vi "Autonomous Independent.vi"() -> ()   [LabVIEW 2018]
doc: "This VI is called when autonomous begins, and will automatically be terminated when autonomous ends. You can carry out timed or sensor driven robot movement independently without needing to return to the caller."
uses:
  <vilib>/Rock Robotics/WPI/RobotDrive/WPI_RobotDriveArcadeDrive_Standard(NoSaturation).vi
  <vilib>/Rock Robotics/Network Tables/NT Write Numeric Array.vi
  <vilib>/Rock Robotics/WPI/Gyro/WPI_GyroXRS450_SPI_Open.vi
  <vilib>/Rock Robotics/Network Tables/NT Write Number.vi
  <vilib>/Rock Robotics/Network Tables/NT Read String.vi
  <vilib>/Rock Robotics/SystemInterfaces/spilib/spi_bus.ctl
panel:
  out "Ultrasonic 2":dbl
  out "Ultrasonic":dbl
  out "Degrees 2":dbl(knob) scale=0.0..360.0
  out "Degrees":dbl(knob) scale=0.0..360.0
  in  "Reset Angle?":bool
  out "Calibrated?":bool
  out "Degrees":dbl(knob) scale=0.0..360.0
  out "Degrees 2":dbl(knob) scale=0.0..360.0
  in  "SPI Bus":T1
  out "Device Found":bool
  in  "Sample Rate (Hz)":dbl=1000.0 min=50.0 max=20000.0 format="%#_13g"
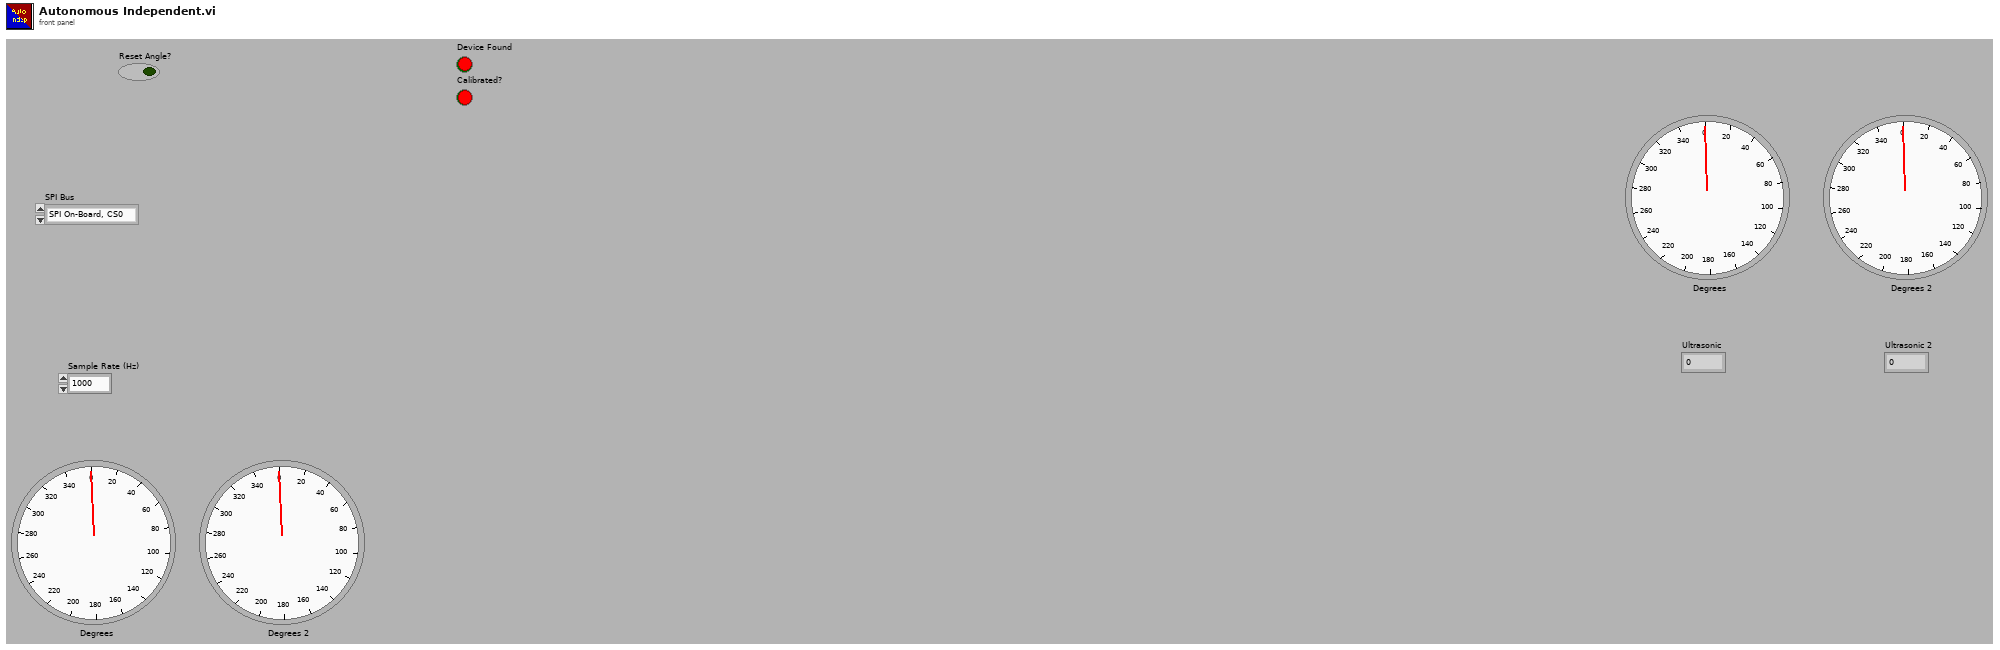
[diagram p1: front panel]
types:
  T1 = typedef "spi_bus.ctl" = enum16{"SPI On-Board, CS0", "SPI On-Board, CS1", "SPI On-Board, CS2", "SPI On-Board, CS3", "SPI MXP", "Invalid"}
  T2 = typedef "WPI_JoystickDevRef.ctl" = cluster{"Device":T3}
  T3 = typedef "WPI_JoystickDeviceEnum.ctl" = enum16{"USB 0", "USB 1", "USB 2", "USB 3", "USB 4", "USB 5"}
  T4 = typedef "WPI_RobotDriveDevRef.ctl" = cluster{"DevStatus":errorcluster, "Motors[]":T5[], "Square Inputs":bool, "Max Output":dbl}
  T5 = typedef "WPI_MotorControlDeviceRef.ctl" = cluster{"DeviceStatus":errorcluster, "Type":T6, "PWM":cluster{"PWM Channel":T7, "DeadBand":T8}, "CAN":cluster{"Device Number":u8, "SetOutput VI Ref":variant, "GetOutput VI Ref":variant, "Enable VI Ref":variant, "Disable VI Ref":variant, "Data":variant}, "Invert":bool, "DIO PWM":cluster{"PWM \"Enable\" Channel":T7, "DIOChannel":T9, "PWM Rate":dbl}}
  T6 = typedef "WPI_MotorControlType.ctl" = enum16{"PWM", "CAN", "DIO PWM"}
  T7 = typedef "FPGA_DIOPWMChannel.ctl" = enum8{"PWM 0", "PWM 1", "PWM 2", "PWM 3", "PWM 4", "PWM 5", "PWM 6", "PWM 7", "PWM 8", "PWM 9", "PWM MXP 0", "PWM MXP 1", "PWM MXP 2", "PWM MXP 3", "PWM MXP 4", "PWM MXP 5", "PWM MXP 6", "PWM MXP 7", "PWM MXP 8", "PWM MXP 9", "Invalid"}
  T8 = typedef "WPI_PWMDeadband.ctl" = cluster{"Name":string, "maxPositivePwm":i32, "minPositivePwm":i32, "centerPwm":i32, "maxNegativePwm":i32, "minNegativePwm":i32, "angularRange":u16}
  T9 = typedef "FPGA_DIOChannel.ctl" = enum8{"DIO 0", "DIO 1", "DIO 2", "DIO 3", "DIO 4", "DIO 5", "DIO 6", "DIO 7", "DIO 8", "DIO 9", "DIO MXP 0", "DIO MXP 1", "DIO MXP 2", "DIO MXP 3", "DIO MXP 4", "DIO MXP 5", "DIO MXP 6", "DIO MXP 7", "DIO MXP 8", "DIO MXP 9", "DIO MXP 10", "DIO MXP 11", "DIO MXP 12", "DIO MXP 13", "DIO MXP 14", "DIO MXP 15", "SPI Port CS1", "SPI Port CS2", "SPI Port CS3", "SPI Port MISO", "SPI Port MOSI", "Invalid"}
  T10 = typedef "WPI_GyroDevRef.ctl" = cluster{"DevStatus":errorcluster, "Analog Channel":T11, "Gain (VoltsPerDegree/Second)":dbl, "Gyro Type":enum16{"Analog", "XRS450"}, "Handle":i32, "SPI Bus":T1, "Device Found":bool, "Sample Rate":dbl, "Calibrate On Open":bool, "Offset":dbl}
  T11 = typedef "FPGA_AIChannel.ctl" = enum8{"AI 0", "AI 1", "AI 2", "AI 3", "AI MXP 0", "AI MXP 1", "AI MXP 2", "AI MXP 3", "Invalid"}
  T12 = typedef "WPI_AnalogChannelDevRef.ctl" = cluster{"DevStatus":errorcluster, "Analog Channel":T11}
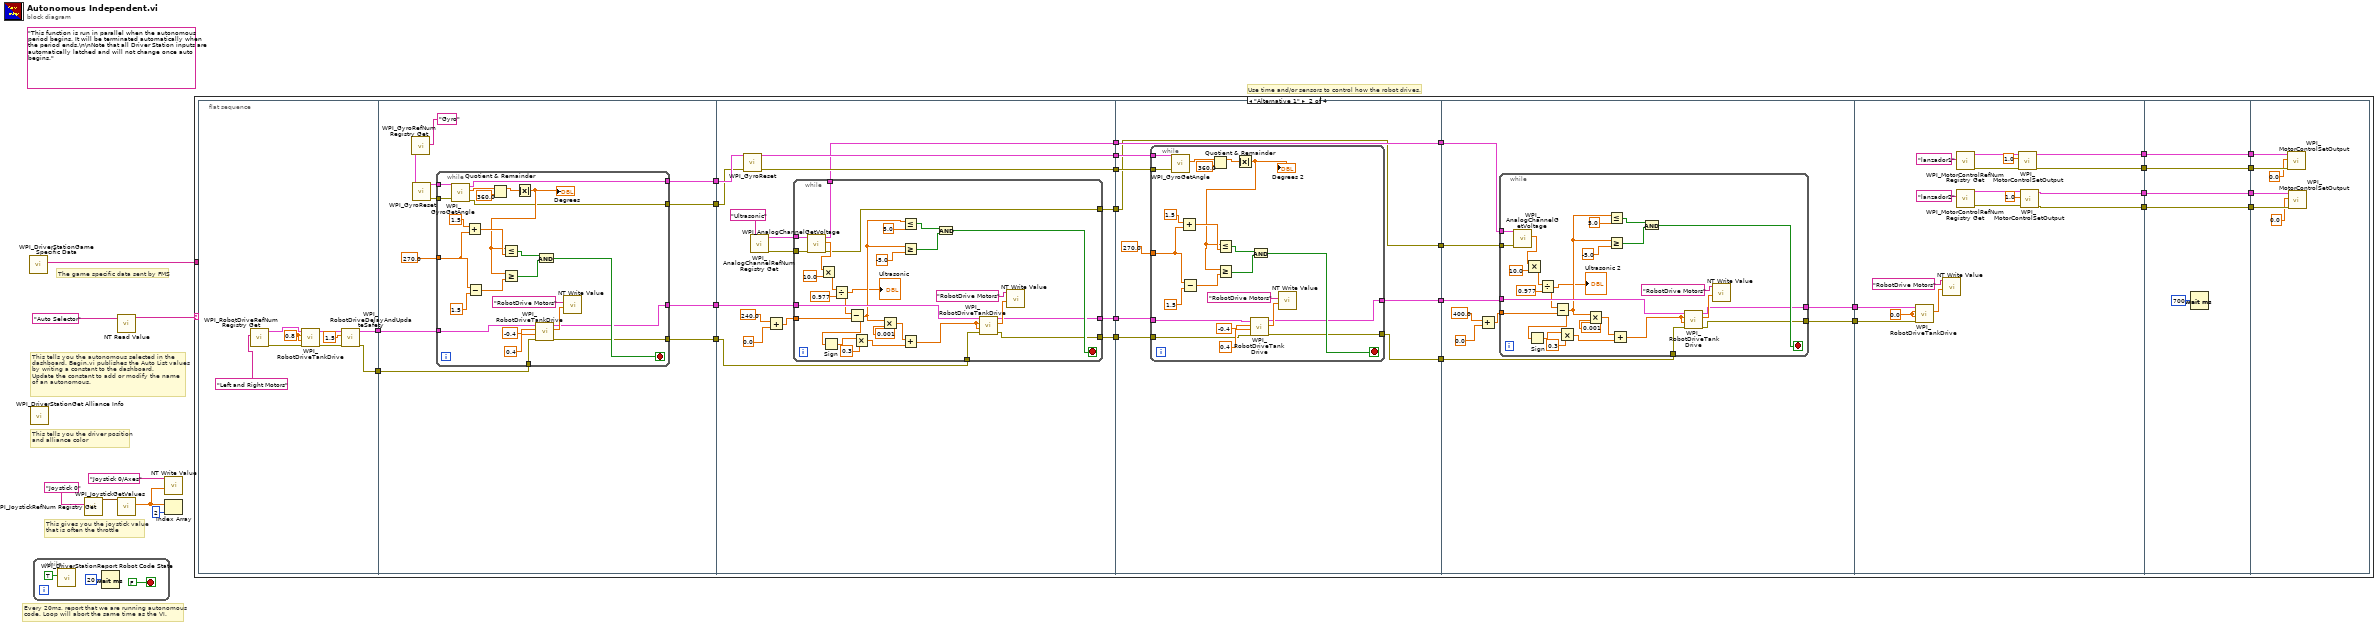
[diagram p0: block diagram]
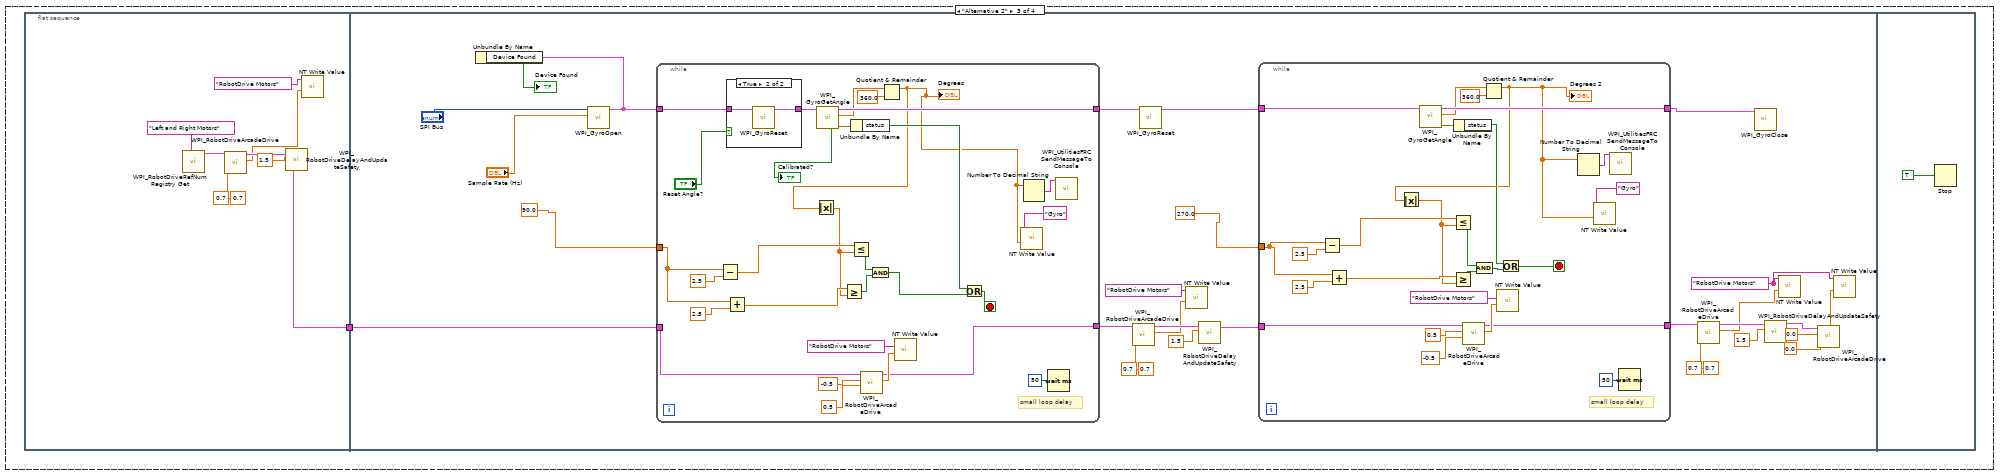
[diagram p3: hidden frame]
diagram:
  (unwired) "This function is run in parallel when the autonomous period begins. It will be terminated automatically when the period ends.\n\nNote that all Driver Station inputs are automatically latched and will not change once auto begins."
  # "The game specific data sent by FMS"
  # "This tells you the autonomous selected in the \ndashboard. Begin.vi publishes the Auto List values\nby writing a constant to the dashboard.\nUpdate the constant to add or modify the name\nof an autonomous."
  # "Every 20ms, report that we are running autonomous\ncode. Loop will abort the same time as the VI."
  # "This gives you the joystick value\nthat is often the throttle"
  # "Use time and/or sensors to control how the robot drives."
  # "This tells you the driver position\nand alliance color"
  n1 = call <vilib>:"WPI_DriverStationGame Specific Data.vi"() -> ("Game Specific Data"=w1:string)  [unwired: 11 in]
  n2 = call <vilib>:"WPI_DriverStationGet Alliance Info.vi"() -> ()  [unwired: 12 out]
  n3 = while {
    stop <- FALSE stop-if-true
    n4 = call <vilib>:"WPI_DriverStationReport Robot Code State.vi"("Autonomous"=TRUE) -> ()  [unwired: 10 in, 1 out]
    n5 = Wait (ms)(milliseconds to wait=u32 20) -> ()  [unwired: 1 out]
  }
  n6 = call <vilib>:"WPI_JoystickRefNum Registry Get.vi"("refnum name"="Joystick 0") -> ("JoystickDevRef"=w7:T2)  [unwired: 1 in, 9 out]
  n7 = call <vilib>:"WPI_JoystickGetValues.vi"("JoystickDevRef"=w7) -> ("Axes"=w3:dbl[])  [unwired: 6 in, 4 out]
  n8 = call-poly <vilib>:"NT Read Value.vi"("Name"="Auto Selector") -> ("String"=w4:string)  [unwired: 9 in, 1 out]
  n9 = call-poly <vilib>:"NT Write Value.vi"("Numeric Array"=w3, "Name"="Joystick 0/Axes") -> ()  [unwired: 9 in, 1 out]
  n10 = Index Array(array=w3, index=2) -> ()  [unwired: 1 out]
  n11 = case shown="\"Alternative 1\"" w4 {
    tunnel: w1 -> [_ _ _ _]
    frame Default {
      # "You can put your main auto here, or you can right-click on the case and make any\nother frame be the default case."
      # "This is the frame that will execute if no selection is made, or if it is not recognized"
    }
    frame "Alternative 1" {
      n12 = flat-sequence {
        tunnel: [w39] -> w13
        tunnel: [w40] -> w12
        tunnel: [w52] -> w37
        tunnel: [w51] -> w36
        tunnel: [w50] -> w35
        tunnel: [w49] -> w34
        tunnel: w13 -> [w48]
        tunnel: w12 -> [w47]
        tunnel: w37 -> [w92]
        tunnel: w36 -> [w91]
        tunnel: w35 -> [w90]
        tunnel: w34 -> [w89]
        tunnel: [w88] -> w33
        tunnel: [w87] -> w32
        tunnel: [w86] -> w31
        tunnel: [w85] -> w30
        tunnel: [w84] -> w26
        tunnel: [w83] -> w24
        tunnel: w33 -> [w135]
        tunnel: w32 -> [w134]
        tunnel: w31 -> [w132]
        tunnel: w30 -> [w131]
        tunnel: [w130] -> w29
        tunnel: [w129] -> w28
        tunnel: [w128] -> w27
        tunnel: w26 -> [w128]
        tunnel: [w127] -> w25
        tunnel: w24 -> [w127]
        tunnel: w29 -> [w166]
        tunnel: w28 -> [w162]
        tunnel: w27 -> [w161]
        tunnel: w25 -> [w160]
        tunnel: [w159] -> w23
        tunnel: [w158] -> w22
        tunnel: w23 -> [w199]
        tunnel: w22 -> [w198]
        tunnel: [w196] -> w20
        tunnel: [w195] -> w18
        tunnel: [w194] -> w16
        tunnel: [w193] -> w14
        tunnel: [w213] -> w21
        tunnel: w20 -> [w213]
        tunnel: [w212] -> w19
        tunnel: w18 -> [w212]
        tunnel: [w211] -> w17
        tunnel: w16 -> [w211]
        tunnel: [w210] -> w15
        tunnel: w14 -> [w210]
        tunnel: w21 -> [w220]
        tunnel: w19 -> [w219]
        tunnel: w17 -> [w218]
        tunnel: w15 -> [w217]
        frame #0 {
          w46 = 0.8 ("Left axis value")
          n13 = call <vilib>:"WPI_RobotDriveRefNum Registry Get.vi"("refnum name"="Left and Right Motors") -> ("error out"=w44:errorcluster, "RobotDriveDevRef"=w45:T4)  [unwired: 9 in]
          n14 = call <vilib>:"WPI_RobotDriveTankDrive.vi"("error in (no error)"=w44, "Right axis value"=w46, "Left axis value"=w46, "RobotDriveDevRef"=w45) -> ("error out"=w42:errorcluster, "RobotDriveDevRef"=w43:T4)  [unwired: 5 in, 1 out]
          n15 = call <vilib>:"WPI_RobotDriveDelayAndUpdateSafety.vi"("error in (no error)"=w42, "Delay (s)"=1.5, "RobotDriveDevRef"=w43) -> ("error out"=w39:errorcluster, "RobotDriveDevRef 2"=w40:T4)  [unwired: 7 in]
        }
        frame #1 {
          n16 = call <vilib>:"WPI_GyroRefNum Registry Get.vi"("refnum name"="Gyro") -> ("error out"=w56:errorcluster, "GyroDevRef"=w57:T10)  [unwired: 9 in]
          n17 = call <vilib>:"WPI_GyroReset.vi"("error in"=w56, "GyroDevRef"=w57) -> ("error out"=w54:errorcluster, "GyroDevRef"=w55:T10)  [unwired: 8 in]
          n18 = while {
            tunnel: w55 -> [w82]
            tunnel: w54 -> [w81]
            tunnel: 270.0 ("y") -> [w73]
            tunnel: [w64] -> w52
            tunnel: [w63] -> w51
            tunnel: [w62] -> w50
            tunnel: [w61] -> w49
            tunnel: w48 -> [w60]
            tunnel: w47 -> [w59]
            stop <- w76 stop-if-true
            n19 = call <vilib>:"WPI_GyroGetAngle.vi"("error in"=w81, "GyroDevRef"=w82) -> ("error out"=w61:errorcluster, "Angle"=w68:dbl, "GyroDevRef"=w62:T10)  [unwired: 5 in, 2 out]
            n20 = Add(x=1.5 ("y"), y=w73) -> (x+y=w69:dbl)
            n21 = Subtract(x=w73, y=1.5 ("x")) -> (x-y=w70:dbl)
            n22 = Quotient & Remainder(x=w68, y=360.0) -> (x-y*floor(x/y)=w66:dbl)  [unwired: 1 out]
            n23 = Absolute Value(x=w66) -> (abs(x)=w65:dbl)
            "Degrees" <- w65
            n24 = Less Or Equal?(x=w65, y=w69) -> (x <= y?=w71:bool)
            n25 = Greater Or Equal?(x=w65, y=w70) -> (x >= y?=w72:bool)
            n26 = call <vilib>:"WPI_RobotDriveTankDrive.vi"("error in (no error)"=w60, "Right axis value"=0.4 ("X axis value"), "Left axis value"=-0.4 ("X axis value"), "RobotDriveDevRef"=w59) -> ("error out"=w63:errorcluster, "Motor Values"=w80:dbl[], "RobotDriveDevRef"=w64:T4)  [unwired: 5 in]
            n27 = And(x=w71, y=w72) -> (x .and. y?=w76:bool)
            n28 = call-poly <vilib>:"NT Write Value.vi"("Numeric Array"=w80, "Name"="RobotDrive Motors") -> ()  [unwired: 9 in, 1 out]
          }
        }
        frame #2 {
          n29 = call <vilib>:"WPI_GyroReset.vi"("error in"=w89, "GyroDevRef"=w90) -> ("error out"=w85:errorcluster, "GyroDevRef"=w86:T10)  [unwired: 8 in]
          n30 = call <vilib>:"WPI_AnalogChannelRefNum Registry Get.vi"("refnum name"="Ultrasonic") -> ("error out"=w97:errorcluster, "AIDeviceRef"=w96:T12)  [unwired: 9 in]
          n31 = Add(x=240.0 ("y"), y=0.0) -> (x+y=w93:dbl)
          n32 = while {
            tunnel: w97 -> [w122]
            tunnel: w96 -> [w121]
            tunnel: w93 -> [w120]
            tunnel: w92 -> [w115]
            tunnel: w91 -> [w111]
            tunnel: [w103] -> w88
            tunnel: [w102] -> w87
            tunnel: [w100] -> w84
            tunnel: [w99] -> w83
            stop <- w107 stop-if-true
            n33 = call <vilib>:"WPI_AnalogChannelGetVoltage.vi"("error in (no error)"=w122, "AIDeviceRef"=w121) -> ("error out"=w99:errorcluster, "Voltage"=w125:dbl, "AIDeviceRef"=w100:T12)  [unwired: 7 in]
            n34 = Multiply(x=w125, y=10.0) -> (x*y=w126:dbl)
            n35 = Divide(x=w126, y=0.977) -> (x/y=w101:dbl)
            "Ultrasonic" <- w101
            n36 = Subtract(x=w101, y=w120) -> (x-y=w104:dbl)
            n37 = Sign(1:w104) -> (0:w114:dbl)
            n38 = Multiply(x=w114, y=0.3) -> (x*y=w112:dbl)
            n39 = Multiply(x=w104, y=0.001) -> (x*y=w118:dbl)
            n40 = Less Or Equal?(x=w104, y=5.0 ("x")) -> (x <= y?=w109:bool)
            n41 = Greater Or Equal?(x=w104, y=-5.0 ("x")) -> (x >= y?=w108:bool)
            n42 = Add(x=w118, y=w112) -> (x+y=w110:dbl)
            n43 = And(x=w109, y=w108) -> (x .and. y?=w107:bool)
            n44 = call <vilib>:"WPI_RobotDriveTankDrive.vi"("error in (no error)"=w111, "Right axis value"=w110, "Left axis value"=w110, "RobotDriveDevRef"=w115) -> ("error out"=w103:errorcluster, "Motor Values"=w117:dbl[], "RobotDriveDevRef"=w102:T4)  [unwired: 5 in]
            n45 = call-poly <vilib>:"NT Write Value.vi"("Numeric Array"=w117, "Name"="RobotDrive Motors") -> ()  [unwired: 9 in, 1 out]
          }
        }
        frame #3 {
          n46 = while {
            tunnel: w134 -> [w153]
            tunnel: w135 -> [w152]
            tunnel: 270.0 ("y") -> [w148]
            tunnel: [w140] -> w130
            tunnel: [w139] -> w129
            tunnel: w132 -> [w136]
            tunnel: w131 -> [w137]
            stop <- w151 stop-if-true
            n47 = call <vilib>:"WPI_GyroGetAngle.vi"("error in"=w137, "GyroDevRef"=w136) -> ("Angle"=w143:dbl)  [unwired: 5 in, 4 out]
            n48 = Add(x=1.5 ("y"), y=w148) -> (x+y=w144:dbl)
            n49 = Subtract(x=w148, y=1.5 ("x")) -> (x-y=w145:dbl)
            n50 = Quotient & Remainder(x=w143, y=360.0) -> (x-y*floor(x/y)=w141:dbl)  [unwired: 1 out]
            n51 = Absolute Value(x=w141) -> (abs(x)=w138:dbl)
            "Degrees 2" <- w138
            n52 = Less Or Equal?(x=w138, y=w144) -> (x <= y?=w146:bool)
            n53 = Greater Or Equal?(x=w138, y=w145) -> (x >= y?=w147:bool)
            n54 = call <vilib>:"WPI_RobotDriveTankDrive.vi"("error in (no error)"=w152, "Right axis value"=0.4 ("X axis value"), "Left axis value"=-0.4 ("X axis value"), "RobotDriveDevRef"=w153) -> ("error out"=w139:errorcluster, "Motor Values"=w157:dbl[], "RobotDriveDevRef"=w140:T4)  [unwired: 5 in]
            n55 = And(x=w146, y=w147) -> (x .and. y?=w151:bool)
            n56 = call-poly <vilib>:"NT Write Value.vi"("Numeric Array"=w157, "Name"="RobotDrive Motors") -> ()  [unwired: 9 in, 1 out]
          }
        }
        frame #4 {
          n57 = Add(x=400.0 ("y"), y=0.0) -> (x+y=w163:dbl)
          n58 = while {
            tunnel: w160 -> [w188]
            tunnel: w161 -> [w187]
            tunnel: w163 -> [w186]
            tunnel: w166 -> [w181]
            tunnel: w162 -> [w177]
            tunnel: [w168] -> w159
            tunnel: [w167] -> w158
            stop <- w173 stop-if-true
            n59 = call <vilib>:"WPI_AnalogChannelGetVoltage.vi"("error in (no error)"=w188, "AIDeviceRef"=w187) -> ("Voltage"=w191:dbl)  [unwired: 7 in, 2 out]
            n60 = Multiply(x=w191, y=10.0) -> (x*y=w192:dbl)
            n61 = Divide(x=w192, y=0.977) -> (x/y=w169:dbl)
            "Ultrasonic 2" <- w169
            n62 = Subtract(x=w169, y=w186) -> (x-y=w170:dbl)
            n63 = Sign(1:w170) -> (0:w180:dbl)
            n64 = Multiply(x=w180, y=0.3) -> (x*y=w178:dbl)
            n65 = Multiply(x=w170, y=0.001) -> (x*y=w184:dbl)
            n66 = Less Or Equal?(x=w170, y=5.0 ("x")) -> (x <= y?=w175:bool)
            n67 = Greater Or Equal?(x=w170, y=-5.0 ("x")) -> (x >= y?=w174:bool)
            n68 = Add(x=w184, y=w178) -> (x+y=w176:dbl)
            n69 = And(x=w175, y=w174) -> (x .and. y?=w173:bool)
            n70 = call <vilib>:"WPI_RobotDriveTankDrive.vi"("error in (no error)"=w177, "Right axis value"=w176, "Left axis value"=w176, "RobotDriveDevRef"=w181) -> ("error out"=w167:errorcluster, "Motor Values"=w183:dbl[], "RobotDriveDevRef"=w168:T4)  [unwired: 5 in]
            n71 = call-poly <vilib>:"NT Write Value.vi"("Numeric Array"=w183, "Name"="RobotDrive Motors") -> ()  [unwired: 9 in, 1 out]
          }
        }
        frame #5 {
          w197 = 0.0 ("Left axis value")
          n72 = call <vilib>:"WPI_RobotDriveTankDrive.vi"("error in (no error)"=w198, "Right axis value"=w197, "Left axis value"=w197, "RobotDriveDevRef"=w199) -> ("Motor Values"=w201:dbl[])  [unwired: 5 in, 2 out]
          n73 = call-poly <vilib>:"NT Write Value.vi"("Numeric Array"=w201, "Name"="RobotDrive Motors") -> ()  [unwired: 9 in, 1 out]
          n74 = call <vilib>:"WPI_MotorControlRefNum Registry Get.vi"("refnum name"="lanzador1") -> ("error out"=w208:errorcluster, "MotorControlDevRef"=w209:T5)  [unwired: 9 in]
          n75 = call <vilib>:"WPI_MotorControlRefNum Registry Get.vi"("refnum name"="lanzador2") -> ("error out"=w204:errorcluster, "MotorControlDevRef"=w205:T5)  [unwired: 9 in]
          n76 = call <vilib>:"WPI_MotorControlSetOutput.vi"("error in (no error)"=w208, "Output"=1.0, "MotorControlDevRef"=w209) -> ("error out"=w193:errorcluster, "MotorControlDevRef"=w196:T5)  [unwired: 6 in, 1 out]
          n77 = call <vilib>:"WPI_MotorControlSetOutput.vi"("error in (no error)"=w204, "Output"=1.0, "MotorControlDevRef"=w205) -> ("error out"=w194:errorcluster, "MotorControlDevRef"=w195:T5)  [unwired: 6 in, 1 out]
        }
        frame #6 {
          n78 = Wait (ms)(milliseconds to wait=u32 700) -> ()  [unwired: 1 out]
        }
        frame #7 {
          n79 = call <vilib>:"WPI_MotorControlSetOutput.vi"("error in (no error)"=w217, "Output"=0.0, "MotorControlDevRef"=w220) -> ()  [unwired: 6 in, 3 out]
          n80 = call <vilib>:"WPI_MotorControlSetOutput.vi"("error in (no error)"=w218, "Output"=0.0, "MotorControlDevRef"=w219) -> ()  [unwired: 6 in, 3 out]
        }
      }
    }
    frame "Alternative 2" {
      n81 = flat-sequence {
        tunnel: [w229] -> w221
        tunnel: w221 -> [w258]
        frame #0 {
          n82 = call <vilib>:"WPI_RobotDriveRefNum Registry Get.vi"("refnum name"="Left and Right Motors") -> ("RobotDriveDevRef"=w227:T4)  [unwired: 1 in, 9 out]
          n83 = call-poly <vilib>:"WPI_RobotDriveArcadeDrive.vi"("Y axis value"=0.7, "X axis value"=0.7, "RobotDriveDevRef"=w227) -> ("Motor Values"=w223:dbl[], "RobotDriveDevRef"=w226:T4)  [unwired: 1 in, 6 out]
          n84 = call <vilib>:"WPI_RobotDriveDelayAndUpdateSafety.vi"("Delay (s)"=1.5, "RobotDriveDevRef"=w226) -> ("RobotDriveDevRef 2"=w229:T4)  [unwired: 8 in, 1 out]
          n85 = call-poly <vilib>:"NT Write Value.vi"("Numeric Array"=w223, "Name"="RobotDrive Motors") -> ()  [unwired: 9 in, 1 out]
        }
        frame #1 {
          w240 = "RobotDrive Motors" ("Name")
          n86 = call-poly <vilib>:"WPI_GyroOpen.vi"("Sample Rate (Hz)"="Sample Rate (Hz)", "SPI Bus"="SPI Bus") -> ("GyroDevRef"=w259:T10)  [unwired: 7 in, 2 out]
          n87 = Unbundle By Name(w259) -> ("Device Found"=→"Device Found":bool)
          n88 = while {
            tunnel: w259 -> [w312]
            tunnel: [w310] -> w252
            tunnel: 90.0 ("Angle 3") -> [w294]
            tunnel: w258 -> [w302]
            tunnel: [w301] -> w253
            stop <- w307 stop-if-true
            # "small loop delay"
            n89 = Subtract(x=w294, y=2.5) -> (x-y=w296:dbl)
            n90 = case shown="True" "Reset Angle?" {
              tunnel: w312 -> [w315 w317]
              tunnel: [w315 w316] -> w311
              frame False {
              }
              frame True {
                n91 = call <vilib>:"WPI_GyroReset.vi"("GyroDevRef"=w317) -> ("GyroDevRef"=w316:T10)  [unwired: 9 in, 1 out]
              }
            }
            n92 = Add(x=w294, y=2.5) -> (x+y=w293:dbl)
            n93 = call <vilib>:"WPI_GyroGetAngle.vi"("GyroDevRef"=w311) -> ("error out"=w308:errorcluster, "Angle"=w309:dbl, "GyroDevRef"=w310:T10, "Calibrated?"=→"Calibrated?":bool)  [unwired: 6 in, 1 out]
            n94 = Unbundle By Name(w308) -> ("status"=w300:bool)
            n95 = call-poly <vilib>:"WPI_RobotDriveArcadeDrive.vi"("Y axis value"=0.5 ("X axis value"), "X axis value"=-0.5, "RobotDriveDevRef"=w302) -> ("Motor Values"=w306:dbl[], "RobotDriveDevRef"=w301:T4)  [unwired: 1 in, 6 out]
            n96 = Quotient & Remainder(x=w309, y=360.0) -> (x-y*floor(x/y)=w286:dbl)  [unwired: 1 out]
            "Degrees" <- w286
            n97 = Absolute Value(x=w286) -> (abs(x)=w292:dbl)
            n98 = Greater Or Equal?(x=w293, y=w292) -> (x >= y?=w290:bool)
            n99 = Less Or Equal?(x=w296, y=w292) -> (x <= y?=w291:bool)
            n100 = And(x=w291, y=w290) -> (x .and. y?=w289:bool)
            n101 = call-poly <vilib>:"NT Write Value.vi"("Numeric Array"=w306, "Name"="RobotDrive Motors") -> ()  [unwired: 9 in, 1 out]
            n102 = Or(x=w300, y=w289) -> (x .or. y?=w307:bool)
            n103 = call-poly <vilib>:"NT Write Value.vi"("Numeric"=w286, "Name"="Gyro") -> ()  [unwired: 9 in, 1 out]
            n104 = Number To Decimal String(number=w286) -> (decimal integer string=w287:string)  [unwired: 1 in]
            n105 = Wait (ms)(milliseconds to wait=u32 50) -> ()  [unwired: 1 out]
            n106 = call <vilib>:"WPI_UtilitiesFRC SendMessageToConsole.vi"("Message"=w287) -> ()  [unwired: 14 in, 1 out]
          }
          n107 = call-poly <vilib>:"WPI_RobotDriveArcadeDrive.vi"("Y axis value"=0.7, "X axis value"=0.7, "RobotDriveDevRef"=w253) -> ("Motor Values"=w243:dbl[], "RobotDriveDevRef"=w256:T4)  [unwired: 1 in, 6 out]
          n108 = call <vilib>:"WPI_GyroReset.vi"("GyroDevRef"=w252) -> ("GyroDevRef"=w251:T10)  [unwired: 9 in, 1 out]
          n109 = call-poly <vilib>:"NT Write Value.vi"("Numeric Array"=w243, "Name"="RobotDrive Motors") -> ()  [unwired: 9 in, 1 out]
          n110 = call <vilib>:"WPI_RobotDriveDelayAndUpdateSafety.vi"("Delay (s)"=1.5, "RobotDriveDevRef"=w256) -> ("RobotDriveDevRef 2"=w250:T4)  [unwired: 8 in, 1 out]
          n111 = while {
            tunnel: w251 -> [w272]
            tunnel: [w283] -> w236
            tunnel: 270.0 ("Angle 4") -> [w268]
            tunnel: w250 -> [w275]
            tunnel: [w274] -> w245
            stop <- w280 stop-if-true
            # "small loop delay"
            n112 = Subtract(x=w268, y=2.5) -> (x-y=w270:dbl)
            n113 = Add(x=w268, y=2.5) -> (x+y=w269:dbl)
            n114 = call <vilib>:"WPI_GyroGetAngle.vi"("GyroDevRef"=w272) -> ("error out"=w281:errorcluster, "Angle"=w282:dbl, "GyroDevRef"=w283:T10)  [unwired: 6 in, 2 out]
            n115 = Unbundle By Name(w281) -> ("status"=w273:bool)
            n116 = call-poly <vilib>:"WPI_RobotDriveArcadeDrive.vi"("Y axis value"=-0.5 ("X axis value"), "X axis value"=0.5, "RobotDriveDevRef"=w275) -> ("Motor Values"=w279:dbl[], "RobotDriveDevRef"=w274:T4)  [unwired: 1 in, 6 out]
            n117 = Quotient & Remainder(x=w282, y=360.0) -> (x-y*floor(x/y)=w260:dbl)  [unwired: 1 out]
            "Degrees 2" <- w260
            n118 = Absolute Value(x=w260) -> (abs(x)=w266:dbl)
            n119 = Less Or Equal?(x=w270, y=w266) -> (x <= y?=w265:bool)
            n120 = Greater Or Equal?(x=w269, y=w266) -> (x >= y?=w264:bool)
            n121 = And(x=w265, y=w264) -> (x .and. y?=w263:bool)
            n122 = call-poly <vilib>:"NT Write Value.vi"("Numeric Array"=w279, "Name"="RobotDrive Motors") -> ()  [unwired: 9 in, 1 out]
            n123 = Or(x=w273, y=w263) -> (x .or. y?=w280:bool)
            n124 = Number To Decimal String(number=w260) -> (decimal integer string=w261:string)  [unwired: 1 in]
            n125 = call-poly <vilib>:"NT Write Value.vi"("Numeric"=w260, "Name"="Gyro") -> ()  [unwired: 9 in, 1 out]
            n126 = call <vilib>:"WPI_UtilitiesFRC SendMessageToConsole.vi"("Message"=w261) -> ()  [unwired: 14 in, 1 out]
            n127 = Wait (ms)(milliseconds to wait=u32 50) -> ()  [unwired: 1 out]
          }
          n128 = call-poly <vilib>:"WPI_RobotDriveArcadeDrive.vi"("Y axis value"=0.7, "X axis value"=0.7, "RobotDriveDevRef"=w245) -> ("Motor Values"=w241:dbl[], "RobotDriveDevRef"=w248:T4)  [unwired: 1 in, 6 out]
          n129 = call <vilib>:"WPI_GyroClose.vi"("GyroDevRef"=w236) -> ()  [unwired: 10 in, 1 out]
          n130 = call <vilib>:"WPI_RobotDriveDelayAndUpdateSafety.vi"("Delay (s)"=1.5, "RobotDriveDevRef"=w248) -> ("RobotDriveDevRef 2"=w244:T4)  [unwired: 8 in, 1 out]
          n131 = call-poly <vilib>:"NT Write Value.vi"("Numeric Array"=w241, "Name"=w240) -> ()  [unwired: 9 in, 1 out]
          n132 = call-poly <vilib>:"WPI_RobotDriveArcadeDrive.vi"("Y axis value"=0.0, "X axis value"=0.0, "RobotDriveDevRef"=w244) -> ("Motor Values"=w239:dbl[])  [unwired: 1 in, 7 out]
          n133 = call-poly <vilib>:"NT Write Value.vi"("Numeric Array"=w239, "Name"=w240) -> ()  [unwired: 9 in, 1 out]
        }
        frame #2 {
          n134 = Stop(stop? (T)=TRUE) -> ()
        }
      }
    }
    frame "Stellar" {
    }
  }
